vi "1. ControlRealTimeEx1.vi"() -> ()   [LabVIEW 2011]
panel:
  in  "location":string(combo)="LB201_A225"
  in  "signalID":string(combo)="61"
  in  "IP Address":string(combo)="130.237.50.30"
  in  "value":dbl=20.0
  out "GetDataPCounter":string[][](array[string])
  out "Real-time CO2 data comming from mote 1001":dbl(graph)
  in  "Password":string
  in  "Username":string
  out "Access to HVAC Msg":errorcluster={"status"=FALSE, "code"=0, "source"="Please Wait ..."}
  out "Actuation Result Msg":string
  out "GetDataPlcs Output 4":string[][](array[string])
  out "GetDataPlcs Output 3":string[][](array[string])
  out "GetDataPlcs Output 2":string[][](array[string])
  out "GetDataPlcs Output 1":string[][](array[string])
  out "GetDataMotes Output 5":string[][](array[string])
  out "GetDataMotes Output 4":string[][](array[string])
  out "GetDataMotes Output 3":string[][](array[string])
  out "GetDataMotes Output 2":string[][](array[string])
  out "GetDataMotes Output 1":string[][](array[string])
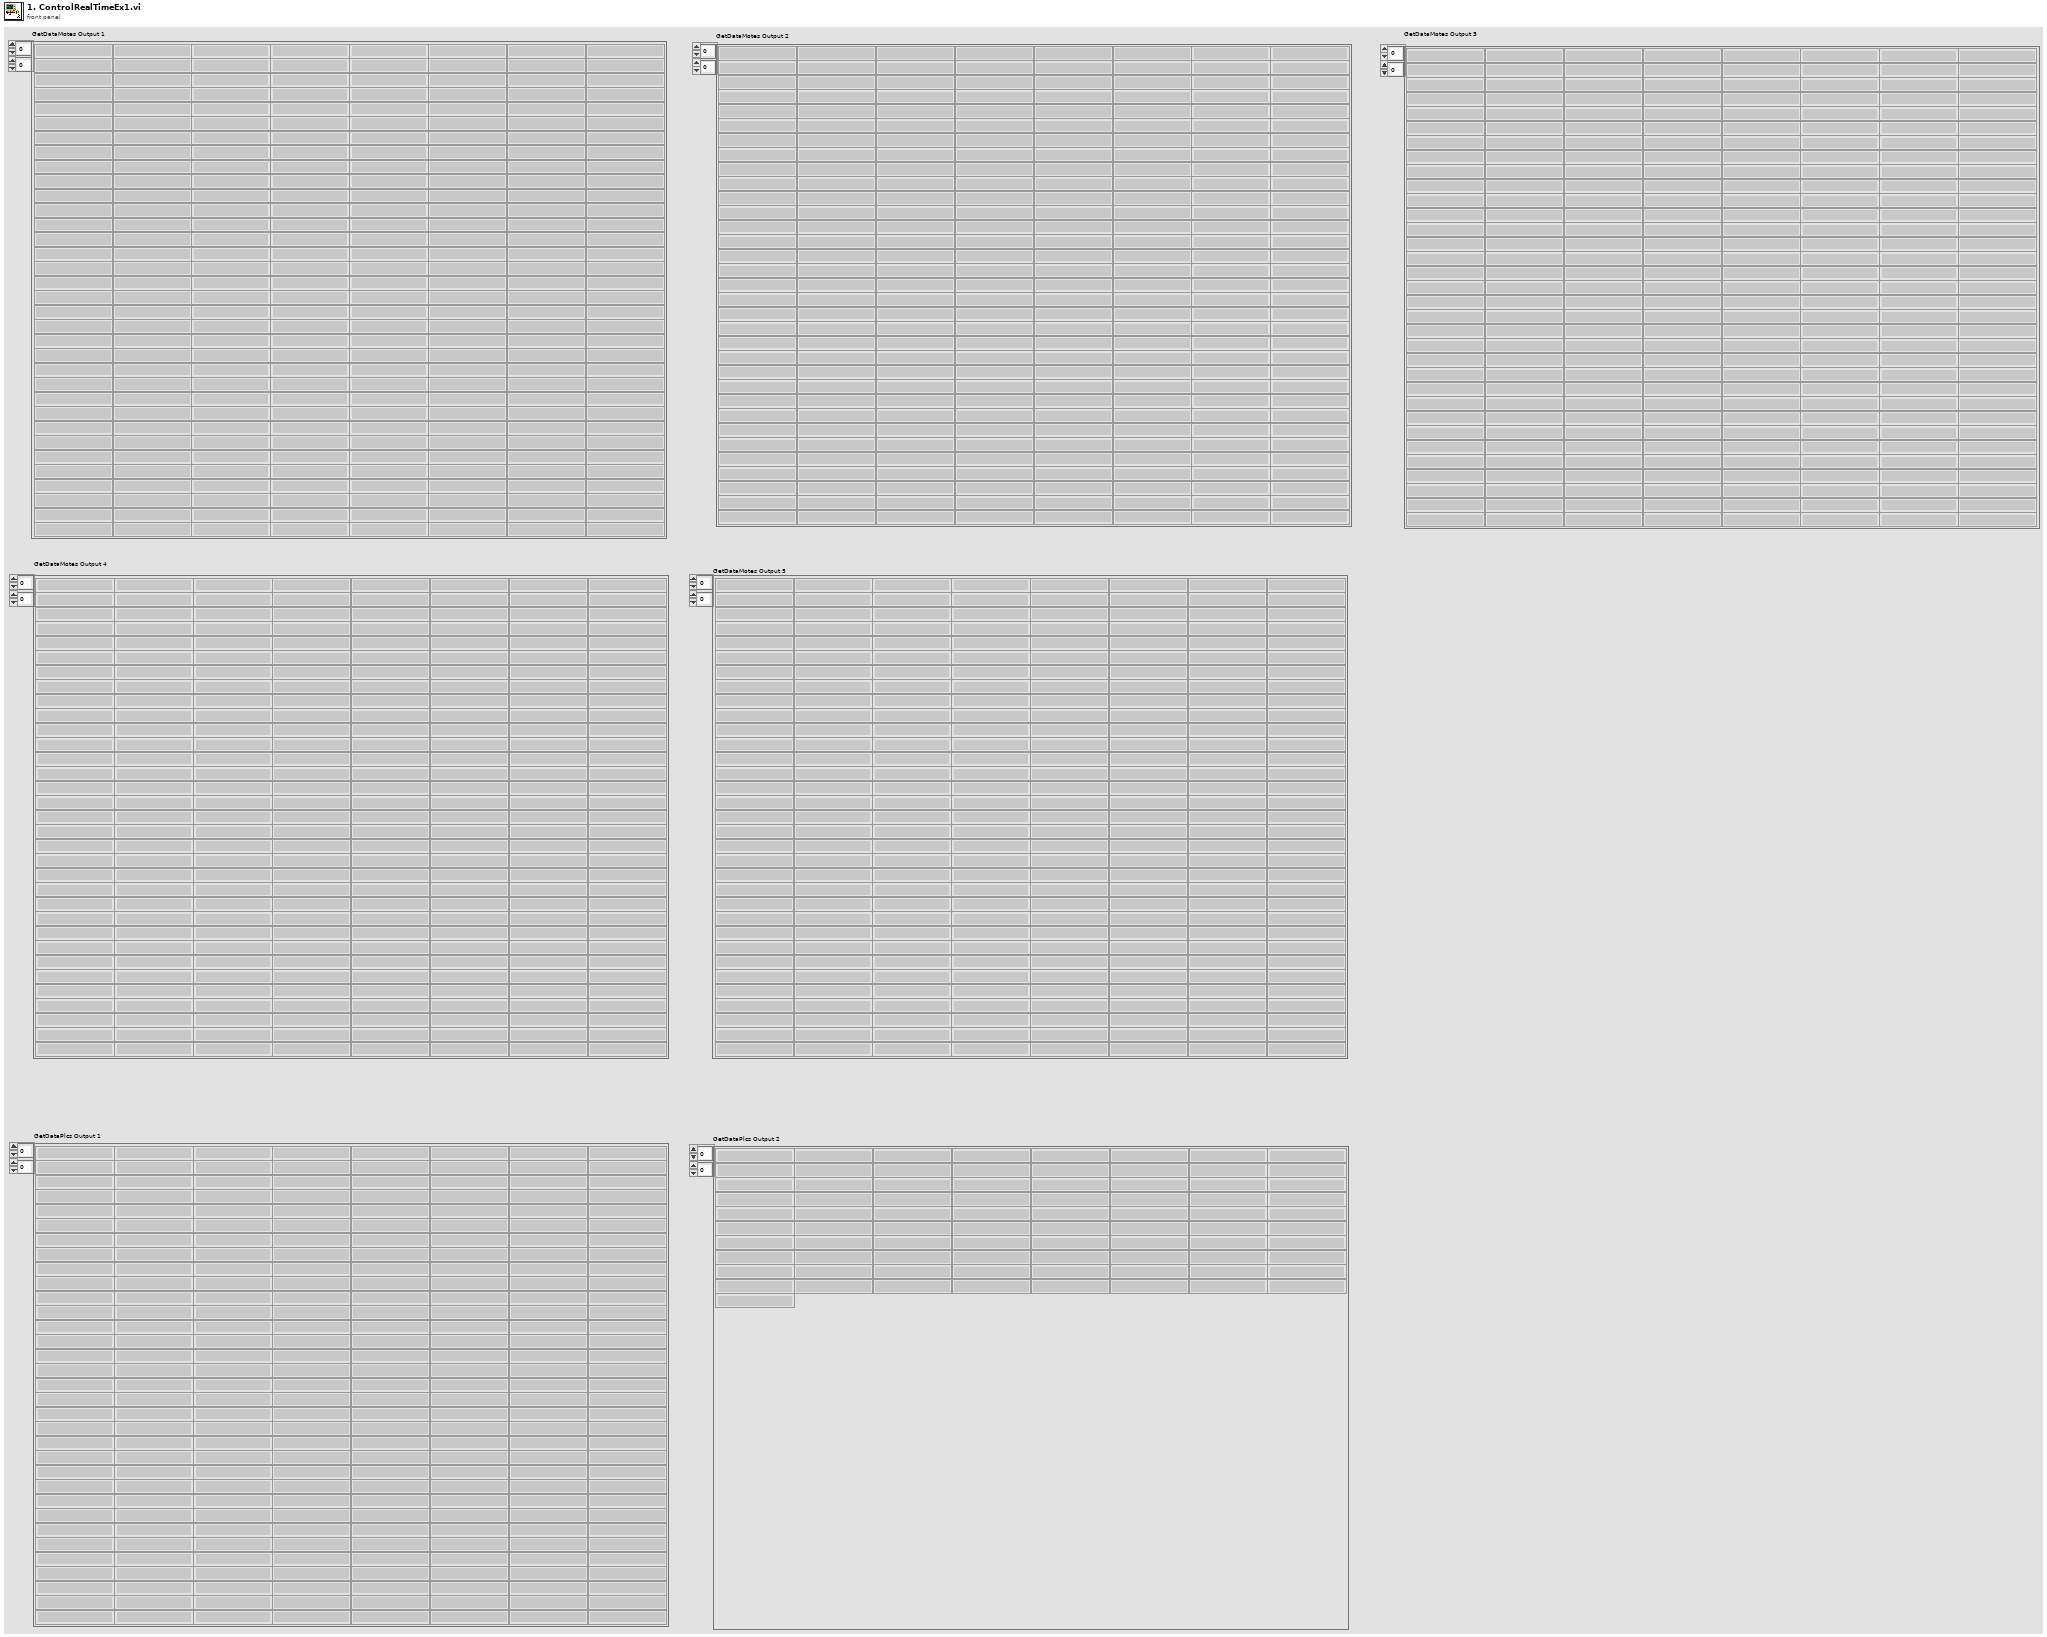
[diagram p1: front panel]
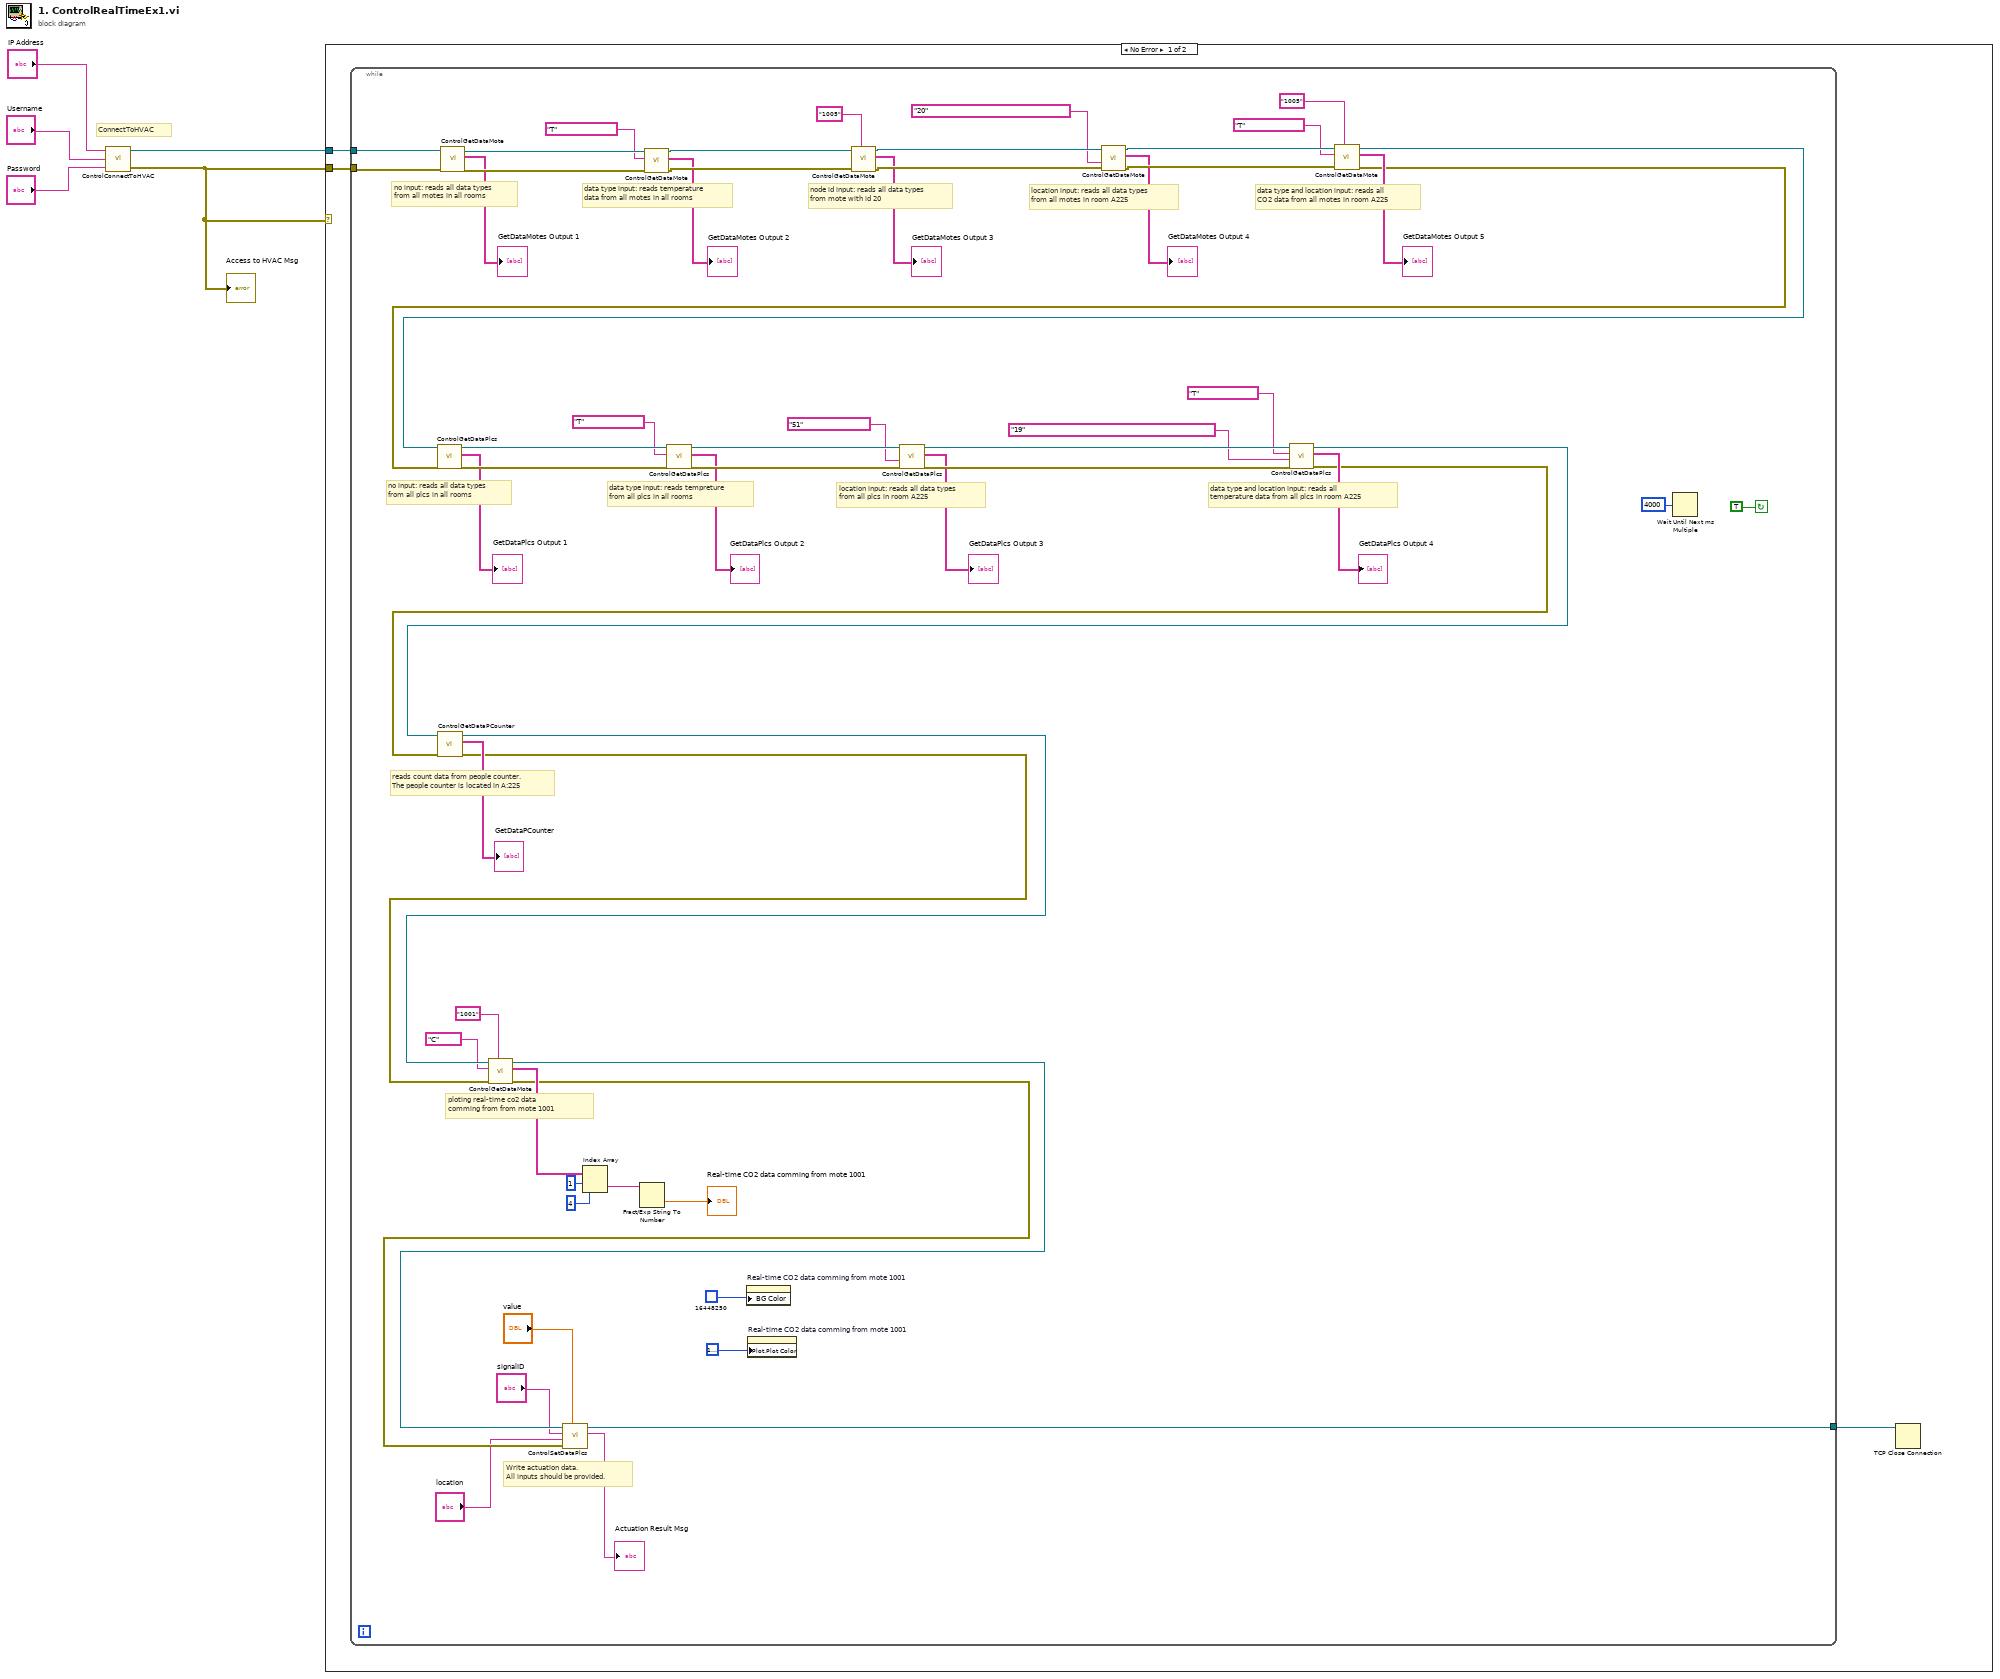
[diagram p0: block diagram]
diagram:
  # "ConnectToHVAC"
  n1 = call "ControlConnectToHVAC.vi"("Password"="Password", "Username"="Username", "IP Address"="IP Address") -> ("error out"=w4:errorcluster, "connection ID out"=w5:refnum<k5>)  [unwired: 1 in]
  "Access to HVAC Msg" <- w4
  n2 = case shown="No Error" w4 {
    tunnel: w5 -> [w8 _]
    tunnel: w4 -> [w7 _]
    frame No Error {
      n3 = while {
        tunnel: w8 -> [w64]
        tunnel: w7 -> [w65]
        tunnel: [w27] -> w6
        stop <- TRUE continue-if-true
        # "Write actuation data. \nAll inputs should be provided."
        # "reads count data from people counter.\nThe people counter is located in A:225"
        # "ploting real-time co2 data \ncomming from from mote 1001"
        # "data type and location input: reads all \ntemperature data from all plcs in room A225"
        # "location input: reads all data types \nfrom all plcs in room A225"
        # "data type input: reads tempreture \nfrom all plcs in all rooms"
        # "no input: reads all data types \nfrom all plcs in all rooms"
        # "data type and location input: reads all \nCO2 data from all motes in room A225"
        # "location input: reads all data types \nfrom all motes in room A225"
        # "node id input: reads all data types\nfrom mote with id 20"
        # "data type input: reads temperature \ndata from all motes in all rooms"
        # "no input: reads all data types \nfrom all motes in all rooms"
        n4 = call "ControlGetDataMote.vi"("error in"=w65, "connection ID in"=w64) -> ("error out"=w56:errorcluster, "output array"=→"GetDataMotes Output 1":string[][], "connection ID out"=w57:refnum<k5>)  [unwired: 7 in]
        n5 = call "ControlGetDataMote.vi"("error in"=w56, "dataType"="T", "connection ID in"=w57) -> ("error out"=w63:errorcluster, "output array"=→"GetDataMotes Output 2":string[][], "connection ID out"=w62:refnum<k5>)  [unwired: 6 in]
        n6 = property on="Real-time CO2 data comming from mote 1001" class="WFChart (strict)"("BG Color"=u32 16448250) -> ()  [unwired: 2 in, 2 out]
        n7 = property on="Real-time CO2 data comming from mote 1001" class="WFChart (strict)"("Plot.Plot Color"=u32 16777222) -> ()  [unwired: 2 in, 2 out]
        n8 = call "ControlGetDataMote.vi"("deviceID"="1005" ("Node ID"), "error in"=w63, "connection ID in"=w62) -> ("error out"=w60:errorcluster, "output array"=→"GetDataMotes Output 3":string[][], "connection ID out"=w61:refnum<k5>)  [unwired: 6 in]
        n9 = call "ControlGetDataMote.vi"("error in"=w60, "signalID"="20", "connection ID in"=w61) -> ("error out"=w58:errorcluster, "output array"=→"GetDataMotes Output 4":string[][], "connection ID out"=w59:refnum<k5>)  [unwired: 6 in]
        n10 = call "ControlGetDataMote.vi"("deviceID"="1005", "error in"=w58, "dataType"="T" ("Data Type"), "connection ID in"=w59) -> ("error out"=w16:errorcluster, "output array"=→"GetDataMotes Output 5":string[][], "connection ID out"=w15:refnum<k5>)  [unwired: 5 in]
        n11 = call "ControlGetDataPlcs.vi"("error in"=w16, "connection ID in"=w15) -> ("error out"=w49:errorcluster, "output array"=→"GetDataPlcs Output 1":string[][], "connection ID out"=w50:refnum<k5>)  [unwired: 6 in]
        n12 = call "ControlGetDataPlcs.vi"("error in"=w49, "dataType"="T", "connection ID in"=w50) -> ("error out"=w48:errorcluster, "output array"=→"GetDataPlcs Output 2":string[][], "connection ID out"=w47:refnum<k5>)  [unwired: 5 in]
        n13 = call "ControlGetDataPlcs.vi"("error in"=w48, "signalID"="51", "connection ID in"=w47) -> ("error out"=w45:errorcluster, "output array"=→"GetDataPlcs Output 3":string[][], "connection ID out"=w46:refnum<k5>)  [unwired: 5 in]
        n14 = call "ControlGetDataPlcs.vi"("error in"=w45, "signalID"="19", "dataType"="T", "connection ID in"=w46) -> ("error out"=w25:errorcluster, "output array"=→"GetDataPlcs Output 4":string[][], "connection ID out"=w24:refnum<k5>)  [unwired: 4 in]
        n15 = call "ControlGetDataPCounter.vi"("error in"=w25, "connection ID in"=w24) -> ("error out"=w30:errorcluster, "output array"=→"GetDataPCounter":string[][], "connection ID out"=w31:refnum<k5>)  [unwired: 7 in]
        n16 = call "ControlGetDataMote.vi"("deviceID"="1001", "error in"=w30, "dataType"="C" ("Data Type"), "connection ID in"=w31) -> ("error out"=w34:errorcluster, "output array"=w39:string[][], "connection ID out"=w35:refnum<k5>)  [unwired: 5 in]
        n17 = call "ControlSetDataPlcs.vi"("data"="value", "error in"=w34, "location"="location", "signalID"="signalID", "connection ID in"=w35) -> ("Output Msg"=→"Actuation Result Msg":string, "connection ID out"=w27:refnum<k5>)  [unwired: 3 in, 1 out]
        n18 = Index Array(array=w39, index (row)=1, index (col)=4 ("disabled index (col)")) -> (element=w36:string)
        n19 = Fract/Exp String To Number(string=w36) -> (number=→"Real-time CO2 data comming from mote 1001":dbl)  [unwired: 3 in, 1 out]
        n20 = Wait Until Next ms Multiple(millisecond multiple=u32 4000) -> ()  [unwired: 1 out]
      }
      n21 = TCP Close Connection(connection ID=w6) -> ()  [unwired: 2 in, 2 out]
    }
    frame Error {
    }
  }
